vi "Add_Row_Times.vi"(3 "Start Index":i32, 5 "Table in":T1[](array[typedef]) {"Carrier_2 Q (l/min)" format="%#.2f"; "Row Duration (mins)" format="%#.1f"; "Row No" min=0; "Trace Gas Concentration (%)" min=0.0 format="%#_4f"; "Carrier_1 Q (l/min)" format="%#.4f"; "Start X" format="%#.2f"; "Start Y" format="%#.2f"; "Start Z" format="%#.2f"; "End X" format="%#.2f"; "End Y" format="%#.2f"; "End Z" format="%#.2f"; "Tunnel Speed" format="%#.2f"; "Averaging time (mins)" min=0.0 format="%#.2f"}) -> (2 "Table Out":T1[](array[typedef]) {"Carrier_2 Q (l/min)" format="%#.2f"; "Row Duration (mins)" format="%#.1f"; "Row No" min=0; "Trace Gas Concentration (%)" min=0.0 format="%#_4f"; "Carrier_1 Q (l/min)" format="%#.4f"; "Start X" format="%#.2f"; "Start Y" format="%#.2f"; "Start Z" format="%#.2f"; "End X" format="%#.2f"; "End Y" format="%#.2f"; "End Z" format="%#.2f"; "Tunnel Speed" format="%#.2f"; "Averaging time (mins)" min=0.0 format="%#.2f"})   [LabVIEW 2020]
uses:
  Controls/Overhead.ctl
  Spacing.ctl
  Controls/Multi_run_mode.ctl
  Traverse_cluster.ctl
panel:
  # "X           Y          Z"
  # "Start"
  # "End"
  # "X           Y          Z"
  # "Start"
  # "End"
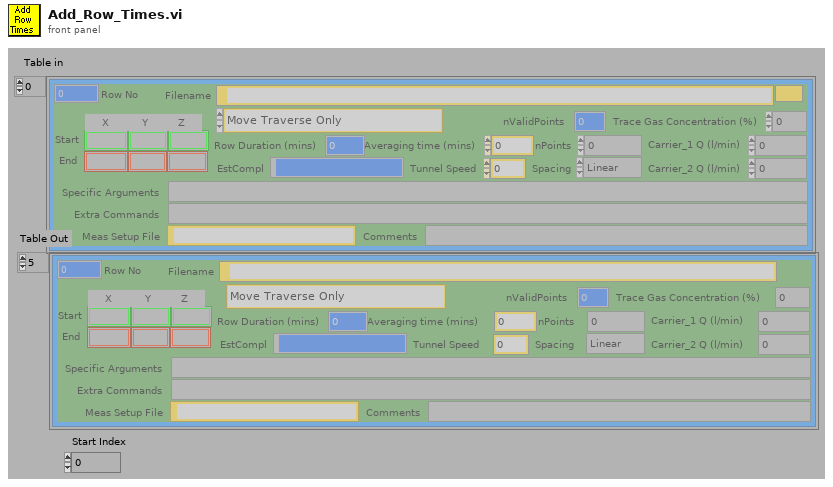
[diagram p1: front panel]
types:
  T1 = typedef "Traverse_cluster.ctl" = cluster{"Start X":sgl, "Start Y":sgl, "Start Z":sgl, "End X":sgl, "End Y":sgl, "End Z":sgl, "nPoints":i32, "Spacing":T2, "Filename":path, "Tunnel Speed":dbl, "Averaging time (mins)":dbl, "Extra Commands":string, "Carrier_1 Q (l/min)":dbl, "Carrier_2 Q (l/min)":dbl, "Trace Gas Concentration (%)":dbl, "Specific Arguments":string, "Comments":string, "Row No":i32, "Row Type Selector":T3, "EstCompl":string, "Row Duration (mins)":dbl, "nValidPoints":i32, "Meas Setup File":string}
  T2 = typedef "Spacing.ctl" = enum16{"Linear", "Log", "Gauss", "Specified", "N/A"}
  T3 = typedef "Multi_run_mode.ctl" = enum16{"Move Traverse Only", "Set Tunnel Speed Only", "Set Source Only", "Set Measurement Conditions", "Single Measurement", "Vertical Profile", "Lateral Profile", "Longitudinal Profile", "Multi-Axis Profile", "Explore Volume", "Auto Calibrate", "Meas Fast FID Bkgnd", "Check Beam Power", "Scanning Valve Measurement", "Run VI Named:", "Set ADAM Ch", "Wait (minutes)", "Send Message", "Synchronize With:", "Fall Back to this Row", "Turn Off Row Repeating", "Traverse 3D Volume", "Blank Row", "Jump to Fall Back Row"}
  T4 = typedef "Overhead.ctl" = enum16{"Update total times", "Read Current Overhead", "Re Scale totals to 3 hrs", "Initialise totals to 3hr"}
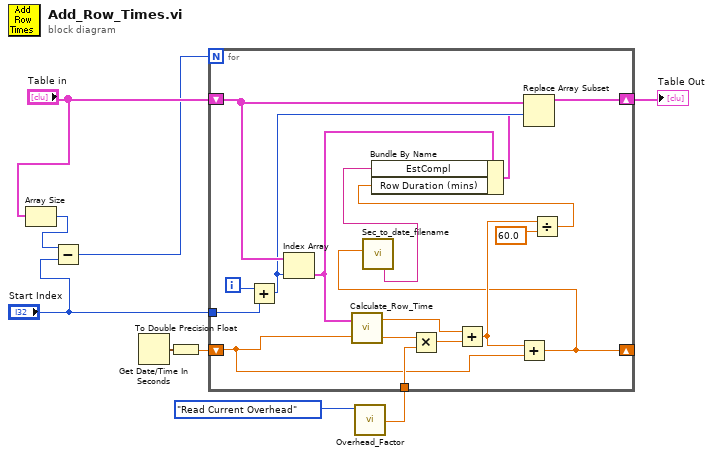
[diagram p0: block diagram]
diagram:
  n1 = Array Size(array="Table in") -> (size(s)=w7:i32)
  n2 = Subtract(x=w7, y="Start Index") -> (x-y=w5:i32)
  n3 = Get Date/Time In Seconds() -> (seconds since 1Jan1904=w1:timestamp)
  n4 = To Double Precision Float(number=w1) -> (double precision float=w4:dbl)
  n5 = call "Overhead_Factor.vi"("Mode"=Overhead."Read Current Overhead") -> ("Current Overhead Factor"=w2:dbl)  [unwired: 3 in]
  n6 = for {
    N: w5 -> [_]
    tunnel: "Start Index" -> [w25]
    shift-right: [w22] -> w9
    shift-left: "Table in" -> [w24]
    shift-right: [w11] -> _
    shift-left: w4 -> [w14]
    tunnel: w2 -> [w20]
    i -> [w26]
    n7 = Add(x=w26, y=w25) -> (x+y=w23:i32)
    n8 = Index Array(array=w24, index=w23) -> (element=w19:T1)
    n9 = call "Calculate_Row_Time.vi"("Multi Run Row"=w19, "Row Start Time (Sec Since 1904)"=w14) -> ("Fixed Time (Sec)"=w17:dbl, "Scalable Time (Sec)"=w21:dbl)  [unwired: 1 out]
    n10 = Multiply(x=w21, y=w20) -> (x*y=w18:dbl)
    n11 = Add(x=w17, y=w18) -> (x+y=w12:dbl)
    n12 = Add(x=w12, y=w14) -> (x+y=w11:dbl)
    n13 = call "Sec_to_date_filename.vi"("ss1904"=w11) -> ("YYYY-mm-DD HH:MM"=w10:string)  [unwired: 5 in, 9 out]
    n14 = Divide(x=w12, y=60.0) -> (x/y=w15:dbl)
    n15 = Bundle By Name(cluster=w19, "EstCompl"=w10, "Row Duration (mins)"=w15) -> (w13:T1)
    n16 = Replace Array Subset(array=w24, new element=w13, index=w23) -> (w22:T1[])
  }
  "Table Out" <- w9
